vi "Create From Quaternion.vi"(8 "error in":errorcluster, 11 "Quaternion":T1) -> (0 "error out":errorcluster, 3 "Orient3d out":refnum<class "Orient3d Class.lvclass">)   [LabVIEW 2017, in "Orient3d Class.lvclass"]
uses:
  Orient3d Class.lvclass
  Type Definitions/Quaternion.ctl
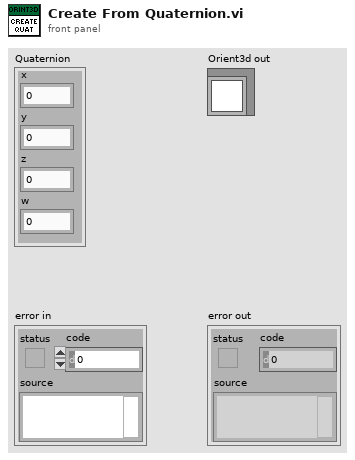
[diagram p1: front panel]
types:
  T1 = typedef "Quaternion.ctl" = cluster{"x":dbl, "y":dbl, "z":dbl, "w":dbl}
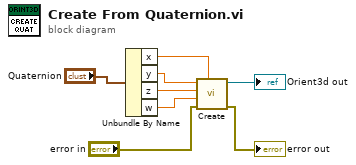
[diagram p0: block diagram]
diagram:
  n1 = Unbundle By Name("Quaternion") -> ("x"=w4:dbl, "y"=w3:dbl, "z"=w2:dbl, "w"=w1:dbl)
  n2 = call "Create.vi"("x"=w4, "error in"="error in", "w"=w1, "z"=w2, "y"=w3) -> ("error out"=→"error out":errorcluster, "Orient3d out"=→"Orient3d out":refnum<class "Orient3d Class.lvclass">)  [unwired: 5 in]
